vi "D触发器设计四人抢答电路.vi"() -> ()   [LabVIEW 2018]
panel:
  in  "结束":bool
  in  "复位":bool
  out "4Q":bool
  out "3Q":bool
  out "2Q":bool
  out "1Q":bool
  in  "4D":bool
  in  "3D":bool
  in  "2D":bool
  in  "1D":bool
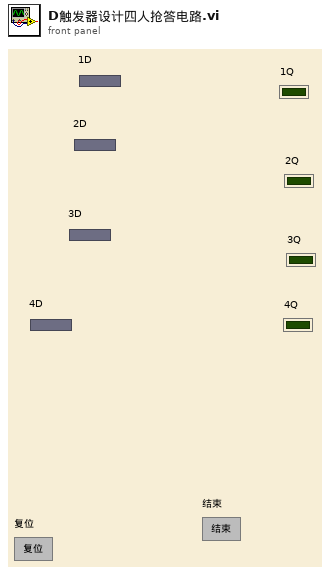
[diagram p1: front panel]
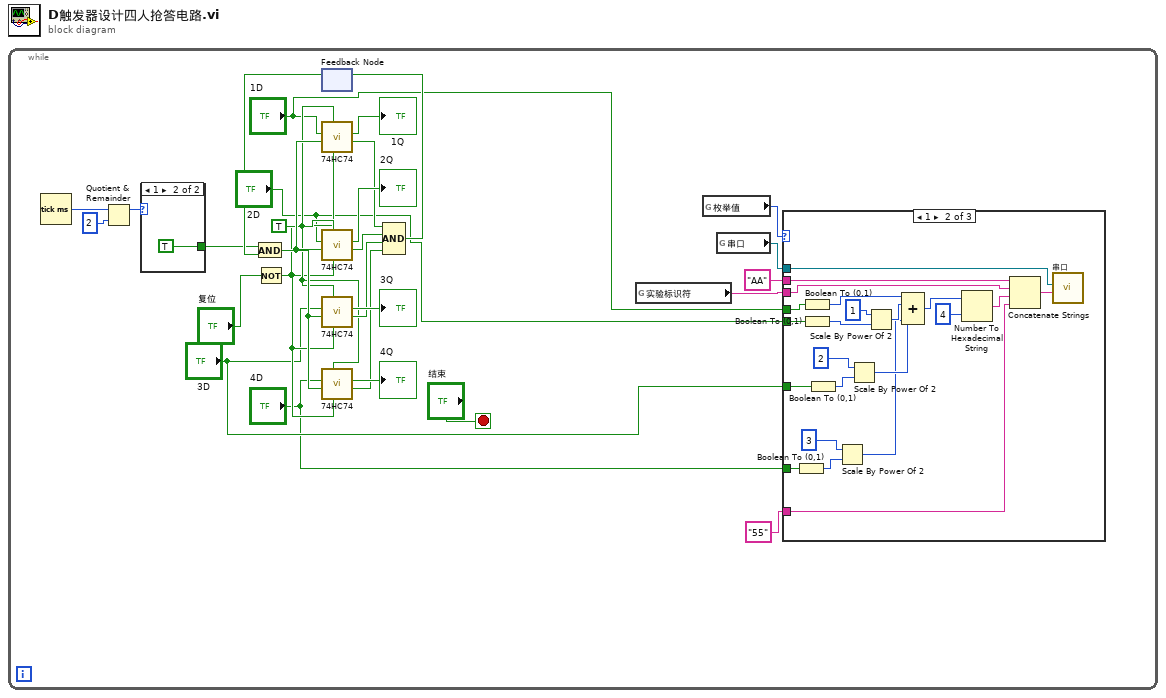
[diagram p0: block diagram]
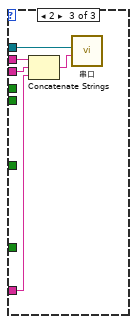
[diagram p3: hidden frame]
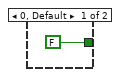
[diagram p4: hidden frame]
diagram:
  n1 = while {
    stop <- "结束" stop-if-true
    w14 = TRUE
    n2 = Tick Count (ms)() -> (millisecond timer value=w22:u32)
    n3 = Quotient & Remainder(x=w22, y=2) -> (x-y*floor(x/y)=w23:u32)  [unwired: 1 out]
    n4 = case shown="1" w23 {
      tunnel: [FALSE TRUE] -> w11
      frame 0, Default {
      }
      frame 1 {
      }
    }
    n5 = Not(x="复位") -> (.not. x?=w12:bool)
    n6 = feedback #1() -> (w15:bool)  [unwired: 1 in]
    n7 = And(x=w11, y=w15) -> (x .and. y?=w21:bool)
    n8 = call "74HC74.vi"("R`"=w12, "S`"=w14, "cp"=w21, "D"="1D") -> ("Q`"=w20:bool, "Q"=→"1Q":bool)  [unwired: 6 in]
    n9 = call "74HC74.vi"("R`"=w12, "S`"=w14, "cp"=w21, "D"="2D") -> ("Q`"=w19:bool, "Q"=→"2Q":bool)  [unwired: 6 in]
    n10 = call "74HC74.vi"("R`"=w12, "S`"=w14, "cp"=w21, "D"="3D") -> ("Q`"=w18:bool, "Q"=→"3Q":bool)  [unwired: 6 in]
    n11 = call "74HC74.vi"("R`"=w12, "S`"=w14, "cp"=w21, "D"="4D") -> ("Q`"=w17:bool, "Q"=→"4Q":bool)  [unwired: 6 in]
    n12 = Compound Arithmetic op=AND ("复合运算")(w20, w19, w18, w17) -> (w16:bool)
    n13 = feedback-in #1(w16) -> ()
    n14 = global read "全局变量.vi" "实验标识符"() -> (w7:string)
    n15 = global read "全局变量.vi" "枚举值"() -> (w9:i8)
    n16 = global read "全局变量.vi" "串口"() -> (w8:refnum<visa-resource-name>)
    n17 = case shown="1" w9 {
      tunnel: w8 -> [_ w45 w53]
      tunnel: w7 -> [_ w44 w54]
      tunnel: "55" -> [_ w43 w51]
      tunnel: "AA" -> [_ w42 w52]
      tunnel: "1D" -> [_ w32 _]
      tunnel: "2D" -> [_ w31 _]
      tunnel: "3D" -> [_ w30 _]
      tunnel: "4D" -> [_ w29 _]
      frame 0, Default {
      }
      frame 1 {
        n18 = Boolean To (0,1)(Boolean=w29) -> (0, 1=w35:i16)
        n19 = Boolean To (0,1)(Boolean=w32) -> (0, 1=w49:i16)
        n20 = Boolean To (0,1)(Boolean=w31) -> (0, 1=w47:i16)
        n21 = Boolean To (0,1)(Boolean=w30) -> (0, 1=w37:i16)
        n22 = Scale By Power Of 2(n=3, x=w35) -> (x*2^n=w33:i16)
        n23 = Scale By Power Of 2(n=2, x=w37) -> (x*2^n=w38:i16)
        n24 = Scale By Power Of 2(n=1, x=w47) -> (x*2^n=w48:i16)
        n25 = Compound Arithmetic op=ADD ("复合运算")(w49, w48, w38, w33) -> (w41:i16)
        n26 = Number To Hexadecimal String(1:4, 2:w41) -> (0:w39:string)
        n27 = Concatenate Strings(w42, w44, w39, w43) -> (w50:string)
        n28 = call "串口.vi"("字符串"=w50, "VISA resource name"=w45) -> ()  [unwired: 10 in]
      }
      frame 2 {
        n29 = Concatenate Strings(w52, w54, w51) -> (w55:string)
        n30 = call "串口.vi"("字符串"=w55, "VISA resource name"=w53) -> ()  [unwired: 10 in]
      }
    }
  }
